vi "MoveAxes.vi"(0 "GoTo Array (Eng units all channels)":T5[](array[typedef]) {"Go To Position" step=100000.0}, 1 "Current Pulses In":dbl[](array[numeric]), 2 "Matched Configurations":T4(array[cluster]) {"Static Drive Configuration"."Indexer Mode  (FSA)" items=["Incremental", "Absolute"]; "Static Drive Configuration"."Buffer at Stop (SSH)" items=["Clear buffer", "Save and Continue"]; "Static Drive Configuration"."Buffer at Limit (SSG)" items=["Clear buffer", "Save and Continue"]; "Static Drive Configuration"."RS232 Echo Control (SSA)" items=["Echo ON", "Echo OFF"]; "Static Drive Configuration"."Reference edge of Home (OSH)" items=["CW", "CCW"]; "Static Drive Configuration"."Encoder Z for Home (OSD)" items=["Don't use", "Enable"]; "Static Drive Configuration"."Home Switch Sense (OSC)" items=["Normally Open", "Normally Closed"]; "Static Drive Configuration"."Home Position (OSB)" items=["Anywhere in Switch", "Edge of Switch"]; "Static Drive Configuration"."Limit Switch Sense (OSA)" items=["Normally Closed", "Normally Open"]; "Static Drive Configuration"."Limit Disable (LD)" items=["Both Enabled", "CW Disabled", "CCW Disabled", "Both Disabled"]; "Static Drive Configuration"."Stall Detect (FSH)" items=["Disable", "Enable"]; "Static Drive Configuration"."OP2 in Deadband (FSG)" items=["Don't Use", "ACTIVATE"]; "Static Drive Configuration"."Stop on Trigger 3 (FSF)" items=["Ignore", "STOP!"]; "Static Drive Configuration"."Activate OP1 on stall (FSE)" items=["Do not Activate", "ACTIVATE!"]; "Static Drive Configuration"."Stop on Stall (FSD)" items=["Continue", "STOP"]; "Static Drive Configuration"."Position Maintenance (FSC)" items=["Disabled", "Enabled"]; "Static Drive Configuration"."Step Mode  (FSB)" items=["Motor", "Encoder"]; "Static Drive Configuration"."Encoder Resolution (ER)" min=1 max=50000; "Static Drive Configuration"."Dead Band Window (DW)" min=0 max=999999999; "Static Drive Configuration"."Dead Band (DB)" min=0 max=999999999; "Static Drive Configuration"."Correction Gain % (CG)" items=["n/a", "12.5", "25", "37.5", "50", "62.5", "75", "87.5", "100"]; "Channel Properties"."Current Pos" format="%.2f"; "Channel Properties"."Backlash/Eng units" format="%.2f"; "Channel Properties"."Pulses/rev" format="%.2f"; "Channel Properties"."Pos Tolerance" format="%.2f"; "Channel Properties"."Pulses/unit" format="%.2f"; "Channel Properties"."Acc. Min" format="%.2f"; "Channel Properties"."Acc. Max" format="%.2f"; "Channel Properties"."Vel. Min" format="%.2f"; "Channel Properties"."Vel. Max" format="%.2f"; "Channel Properties"."Acc. Default" format="%.2f"; "Channel Properties"."Vel. Default" format="%.2f"}, 3 "Current Pos In":dbl[](array[numeric]) format="%.2f", 4 "Home":T1, 5 "Final move":bool) -> (6 "Current Pulses Out":dbl[](array[numeric]), 7 "Current Pos Out":dbl[](array[numeric]) format="%.2f", 8 "Error String":string)   [LabVIEW 2014]
uses:
  ~subVIs/DriveGotoCluster.ctl
  ~subVIs/DriveProperties.ctl
  ~subVIs/DriveStaticConfig.ctl
  Anemometry/Anemometry Sub Vis/Controls/Home.ctl
  ~subVIs/DriveClusterLower.ctl
  ~subVIs/GenericDriveCommand.ctl
  ~subVIs/DriveConfigGlobal.vi
panel:
  out "Retry number":i32
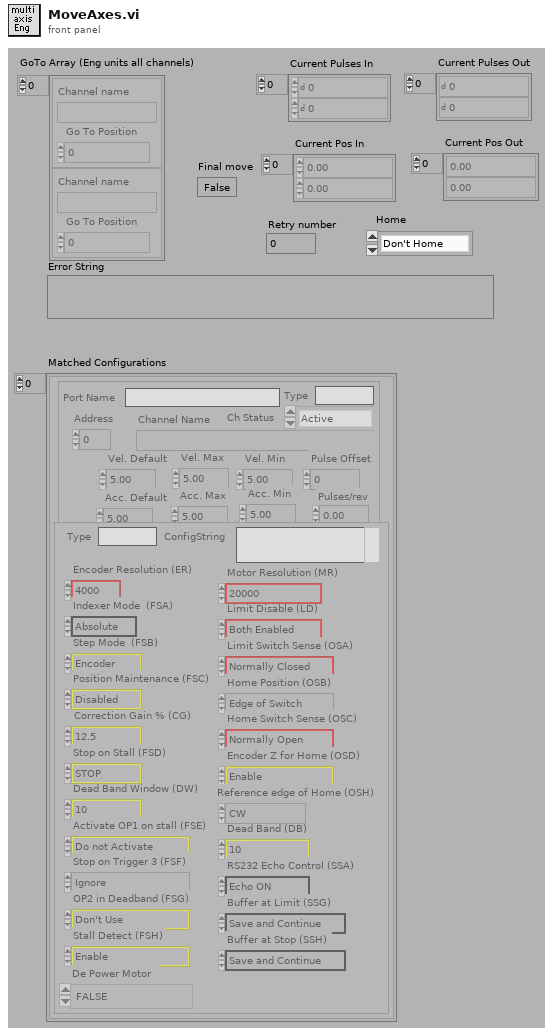
[diagram p1: front panel]
types:
  T1 = typedef "Home.ctl" = enum16{"Don't Home", "Home  +X", "Home  -X", "Home  +Y", "Home  -Y", "Home  +Z", "Home  -Z"}
  T2 = typedef "DriveProperties.ctl" = cluster{"Channel Name":string, "Vel. Default":dbl, "Acc. Default":dbl, "Vel. Max":dbl, "Vel. Min":dbl, "Acc. Max":dbl, "Acc. Min":dbl, "Pulses/unit":dbl, "Address":u8, "Pulse Offset":i32, "Pos Tolerance":dbl, "Pulses/rev":dbl, "Backlash/Eng units":dbl, "Current Pos":dbl, "Ch Status":enum16{"Active", "Offline", "Simulate"}, "Port Name":string, "Axis Transform mode":string, "Metadata Ch Name":string, "Type":string}
  T3 = typedef "DriveStaticConfig.ctl" = cluster{"Correction Gain % (CG)":u16, "Dead Band (DB)":i32, "Dead Band Window (DW)":i32, "Encoder Resolution (ER)":i32, "Step Mode  (FSB)":u16, "Position Maintenance (FSC)":u16, "Stop on Stall (FSD)":u16, "Activate OP1 on stall (FSE)":u16, "Stop on Trigger 3 (FSF)":u16, "OP2 in Deadband (FSG)":u16, "Stall Detect (FSH)":u16, "Limit Disable (LD)":u16, "Motor Resolution (MR)":enum16{"200", "400", "1000", "2000", "4000", "5000", "10000", "12800", "18000", "20000", "21600", "25000", "25400", "25600", "36000", "50000", "278528", "425984", "507904", "614400", "655360", "819200", "1024000"}, "Limit Switch Sense (OSA)":u16, "Home Position (OSB)":u16, "Home Switch Sense (OSC)":u16, "Encoder Z for Home (OSD)":u16, "Reference edge of Home (OSH)":u16, "RS232 Echo Control (SSA)":u16, "Buffer at Limit (SSG)":u16, "Buffer at Stop (SSH)":u16, "Indexer Mode  (FSA)":u16, "Type":string, "ConfigString":string, "De Power Motor":enum16{"TRUE", "FALSE"}}
  T4 = cluster{"Channel Properties":T2, "Static Drive Configuration":T3}[]
  T5 = typedef "DriveGotoCluster.ctl" = cluster{"Channel name":string, "Go To Position":dbl}
  T6 = typedef "GenericDriveCommand.ctl" = string
  T7 = cluster{"Channel Properties":T2, "Static Drive Configuration":T3}
  T8 = cluster{"Total travel time":dbl, "Accelaration time":dbl, "Accelation fractional distance":dbl}
  T9 = typedef "DriveClusterLower.ctl" = cluster{"Go To Position":dbl, "Velocity":dbl, "Acceleration":dbl, "Address":u8}
  T10 = typedef "AxisConfigCluster.ctl" = cluster{"Channel Properties":T2, "Static Drive Configuration":T3}
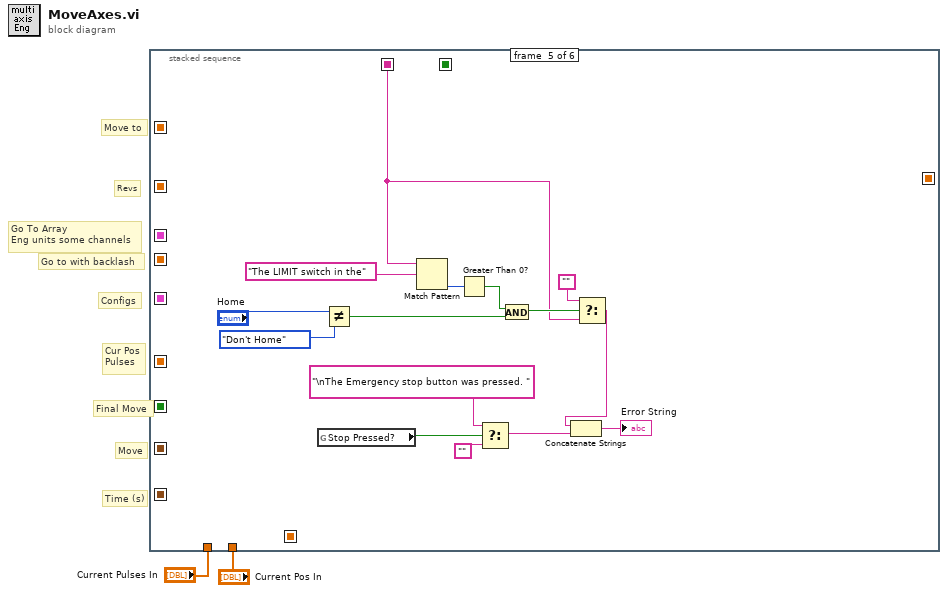
[diagram p0: block diagram]
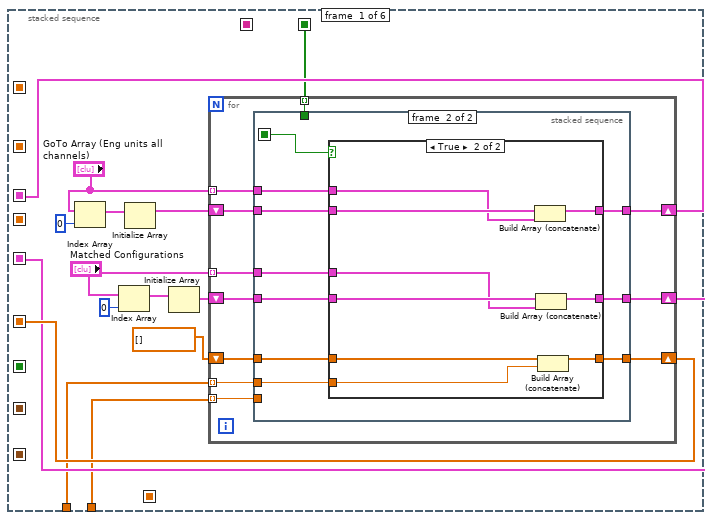
[diagram p2: hidden frame]
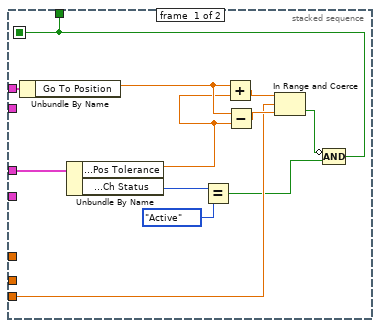
[diagram p3: hidden frame]
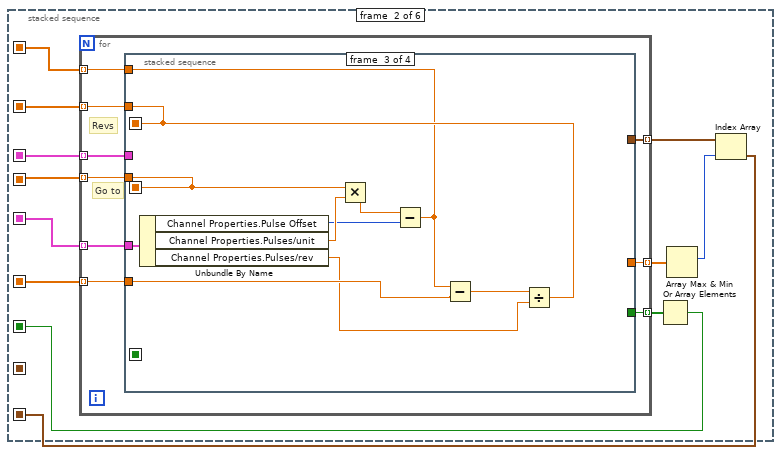
[diagram p5: hidden frame]
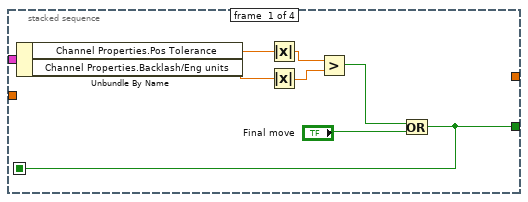
[diagram p6: hidden frame]
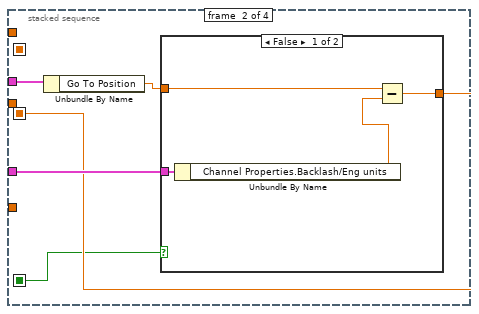
[diagram p7: hidden frame]
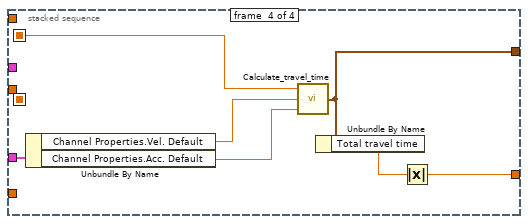
[diagram p9: hidden frame]
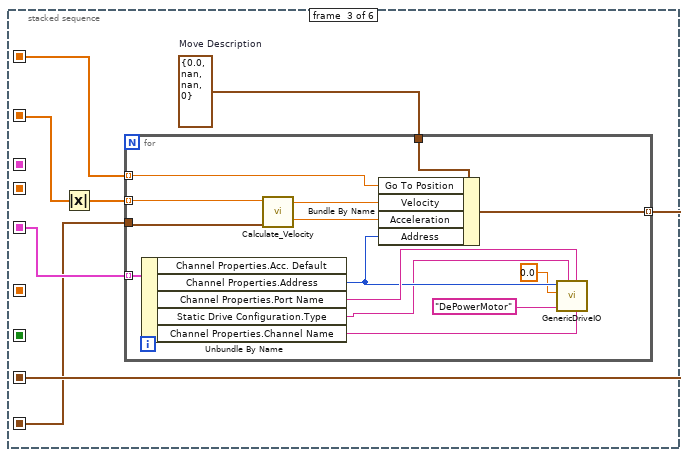
[diagram p10: hidden frame]
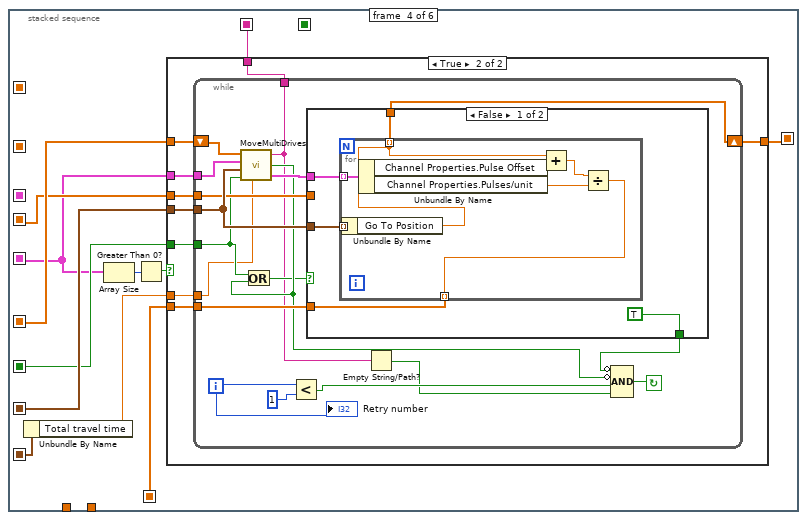
[diagram p11: hidden frame]
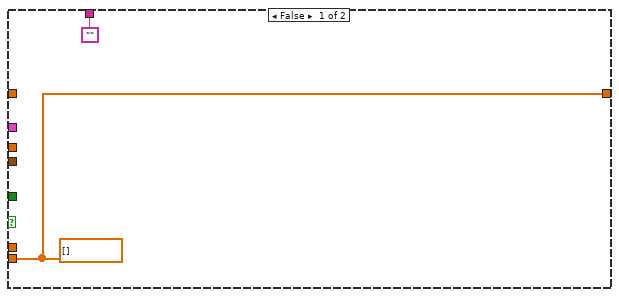
[diagram p12: hidden frame]
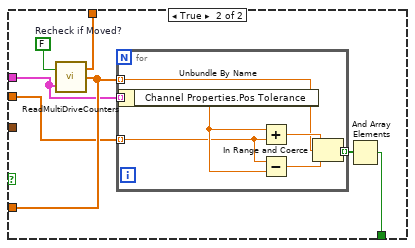
[diagram p13: hidden frame]
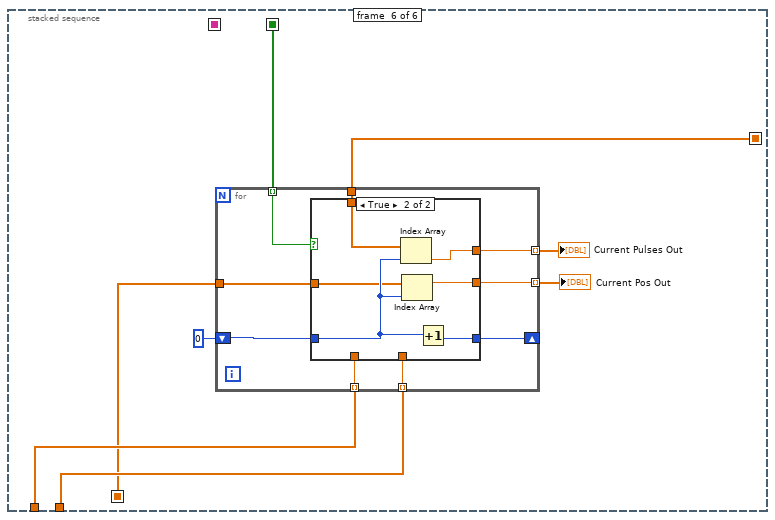
[diagram p14: hidden frame]
diagram:
  # "Go to with backlash"
  # "Final Move"
  # "Move"
  # "Cur Pos\nPulses"
  # "Configs"
  # "Go To Array\nEng units some channels"
  # "Revs"
  # "Move to"
  # "Time (s)"
  n1 = stacked-sequence {
    seq-local: [_ w63 _ _ _ _] -> [_ _ w119 w141 _ _]
    seq-local: [_ w73 _ _ _ _] -> [_ _ w124 _ _ _]
    seq-local: [_ w72 _ _ _ _] -> [_ _ w123 _ _ _]
    seq-local: [w7 _ _ _ _ _] -> [_ w70 _ _ _ _]
    seq-local: [w8 _ _ _ _ _] -> [_ w71 w122 w144 _ _]
    seq-local: [w9 _ _ _ _ _] -> [_ w69 _ w151 _ _]
    seq-local: [_ _ w121 _ _ _] -> [_ _ _ w150 _ _]
    seq-local: [_ _ _ w149 _ _] -> [_ _ _ _ _ w222]
    seq-local: [_ _ _ w148 _ _] -> [_ _ _ _ w212 _]
    seq-local: [w3 _ _ _ _ _] -> [_ _ _ _ _ w228]
    seq-local: [_ _ _ w147 _ _] -> [_ _ _ _ _ w223]
    seq-local: [_ w67 _ _ _ _] -> [_ _ _ w146 _ _]
    seq-local: [_ w66 _ _ _ _] -> [_ _ _ w145 _ _]
    tunnel: "Current Pulses In" -> [w5 _ _ _ _ w227]
    tunnel: "Current Pos In" -> [w4 _ _ _ _ w225]
    frame #0 {
      n2 = Index Array(array="GoTo Array (Eng units all channels)", index=0 ("Index")) -> (element=w15:T5)
      n3 = Index Array(array="Matched Configurations", index=0 ("Index")) -> (element=w13:T7)
      n4 = Initialize Array(w15) -> (w14:T5[])  [unwired: 1 out]
      n5 = Initialize Array(w13) -> (w10:T4)  [unwired: 1 out]
      n6 = for {
        tunnel: "Matched Configurations" -> [w28] mode=indexing
        tunnel: "GoTo Array (Eng units all channels)" -> [w27] mode=indexing
        tunnel: w4 -> [w26] mode=indexing
        shift-right: [w22] -> w7
        shift-left: w14 -> [w23]
        shift-right: [w24] -> w8
        shift-left: w10 -> [w25]
        shift-right: [w20] -> w9
        shift-left: dbl[] [] -> [w21]
        tunnel: w5 -> [w19] mode=indexing
        tunnel: [w18] -> w3 mode=indexing
        n7 = stacked-sequence {
          seq-local: [w33 _] -> [_ w50]
          tunnel: w28 -> [w39 w47]
          tunnel: w27 -> [w40 w44]
          tunnel: w26 -> [w35 _]
          tunnel: w25 -> [_ w49]
          tunnel: [_ w48] -> w24
          tunnel: w23 -> [_ w46]
          tunnel: [_ w45] -> w22
          tunnel: w21 -> [_ w43]
          tunnel: [_ w42] -> w20
          tunnel: w19 -> [_ w41]
          tunnel: [w33 _] -> w18
          frame #0 {
            n8 = Unbundle By Name(w40) -> ("Go To Position"=w38:dbl)
            n9 = Unbundle By Name(w39) -> ("Channel Properties.Pos Tolerance"=w32:dbl, "Channel Properties.Ch Status"=w31:enum16{"Active", "Offline", "Simulate"})
            n10 = Equal?(x=w31, y=enum16{"Active", "Offline", "Simulate"}."Active" ("Channel Properties.Ch Status")) -> (x = y?=w29:bool)
            n11 = Add(x=w38, y=w32) -> (x+y=w37:dbl)
            n12 = Subtract(x=w38, y=w32) -> (x-y=w36:dbl)
            n13 = In Range and Coerce(upper limit=w37, x=w35, lower limit=w36) -> (In Range?=w34:bool)  [unwired: 1 out]
            n14 = Compound Arithmetic op=AND(invert w34, w29) -> (w33:bool)
          }
          frame #1 {
            n15 = case shown="True" w50 {
              tunnel: w49 -> [w52 w62]
              tunnel: [w52 w61] -> w48
              tunnel: w47 -> [_ w60]
              tunnel: w46 -> [w53 w59]
              tunnel: [w53 w58] -> w45
              tunnel: w44 -> [_ w57]
              tunnel: w43 -> [w51 w56]
              tunnel: [w51 w55] -> w42
              tunnel: w41 -> [_ w54]
              frame False {
              }
              frame True {
                n16 = Build Array (concatenate)(w59, w57) -> (w58:T5[])
                n17 = Build Array (concatenate)(w62, w60) -> (w61:T4)
                n18 = Build Array (concatenate)(w56, w54) -> (w55:dbl[])
              }
            }
          }
        }
      }
    }
    frame #1 {
      n19 = for {
        tunnel: w71 -> [w83] mode=indexing
        tunnel: w70 -> [w82] mode=indexing
        tunnel: w69 -> [w81] mode=indexing
        tunnel: [w80] -> w74 mode=indexing
        tunnel: [w79] -> w73 mode=indexing
        tunnel: [w78] -> w72 mode=indexing
        tunnel: [w77] -> w68 mode=indexing
        tunnel: [w76] -> w66 mode=indexing
        tunnel: [w75] -> w65 mode=indexing
        # "Go to"
        # "Revs"
        n20 = stacked-sequence {
          seq-local: [_ _ w108 _] -> [_ _ _ w114]
          seq-local: [_ w93 _ _] -> [_ _ w102 _]
          seq-local: [w84 _ _ _] -> [_ w92 _ _]
          tunnel: w83 -> [w91 w95 w110 w118]
          tunnel: w82 -> [_ w96 _ _]
          tunnel: w81 -> [_ _ w109 _]
          tunnel: [_ _ _ w117] -> w80
          tunnel: [_ _ w105 _] -> w79
          tunnel: [_ _ w108 _] -> w78
          tunnel: [w84 _ _ _] -> w77
          tunnel: [_ _ w102 _] -> w76
          tunnel: [_ _ _ w113] -> w75
          frame #0 {
            n21 = Unbundle By Name(w91) -> ("Channel Properties.Pos Tolerance"=w90:dbl, "Channel Properties.Backlash/Eng units"=w89:dbl)
            n22 = Absolute Value(x=w90) -> (abs(x)=w88:dbl)
            n23 = Absolute Value(x=w89) -> (abs(x)=w87:dbl)
            n24 = Greater?(x=w88, y=w87) -> (0:w86:bool)
            n25 = Or(x=w86, y="Final move") -> (x .or. y?=w84:bool)
          }
          frame #1 {
            n26 = Unbundle By Name(w96) -> ("Go To Position"=w94:dbl)
            n27 = case shown="False" w92 {
              tunnel: w95 -> [w100 _]
              tunnel: w94 -> [w98 w101]
              tunnel: [w97 w101] -> w93
              frame False {
                n28 = Unbundle By Name(w100) -> ("Channel Properties.Backlash/Eng units"=w99:dbl)
                n29 = Subtract(x=w98, y=w99) -> (x-y=w97:dbl)
              }
              frame True {
              }
            }
          }
          frame #2 {
            n30 = Unbundle By Name(w110) -> ("Channel Properties.Pulse Offset"=w103:i32, "Channel Properties.Pulses/unit"=w111:dbl, "Channel Properties.Pulses/rev"=w106:dbl)
            n31 = Multiply(x=w102, y=w111) -> (x*y=w104:dbl)
            n32 = Subtract(x=w104, y=w103) -> (x-y=w105:dbl)
            n33 = Subtract(x=w105, y=w109) -> (x-y=w107:dbl)
            n34 = Divide(x=w107, y=w106) -> (x/y=w108:dbl)
          }
          frame #3 {
            n35 = Unbundle By Name(w118) -> ("Channel Properties.Vel. Default"=w115:dbl, "Channel Properties.Acc. Default"=w116:dbl)
            n36 = call "Calculate_travel_time.vi"("Default Acceleration"=w116, "Default Velocity"=w115, "Revs to travel"=w114) -> ("Times"=w113:T8)
            n37 = Unbundle By Name(w113) -> ("Total travel time"=w112:dbl)
            n38 = Absolute Value(x=w112) -> (abs(x)=w117:dbl)
          }
        }
      }
      n39 = Or Array Elements(Boolean array=w68) -> (logical OR=w67:bool)
      n40 = Array Max & Min(array=w74) -> (max index (indices)=w64:i32)  [unwired: 3 out]
      n41 = Index Array(array=w65, index=w64) -> (element=w63:T8)
    }
    frame #2 {
      w125 = T9 {"Go To Position"=0.0, "Velocity"=nan, "Acceleration"=nan, "Address"=0}  # Move Description
      n42 = Absolute Value(x=w123) -> (abs(x)=w120:dbl[])
      n43 = for {
        tunnel: w125 -> [w139]
        tunnel: w124 -> [w134] mode=indexing
        tunnel: w122 -> [w138] mode=indexing
        tunnel: w120 -> [w135] mode=indexing
        tunnel: [w137] -> w121 mode=indexing
        tunnel: w119 -> [w130]
        n44 = Unbundle By Name(w138) -> ("Channel Properties.Address"=w132:u8, "Channel Properties.Port Name"=w136:string, "Static Drive Configuration.Type"=w128:string, "Channel Properties.Channel Name"=w129:string)  [unwired: 1 out]
        n45 = call "Calculate_Velocity.vi"("Times"=w130, "Revs to travel"=w135) -> ("Acceleration"=w131:dbl, "Max Velocity"=w133:dbl)  [unwired: 1 in, 1 out]
        n46 = Bundle By Name(cluster=w139, "Go To Position"=w134, "Velocity"=w133, "Acceleration"=w131, "Address"=w132) -> (w137:T9)
        n47 = call "GenericDriveIO.vi"("GenericDriveCommand"=T6 "DePowerMotor", "Channel Name"=w129, "Numeric Value"=0.0, "Address"=w132, "Type"=w128, "Port Name"=w136) -> ()  [unwired: 1 in, 5 out]
      }
    }
    frame #3 {
      n48 = Unbundle By Name(w141) -> ("Total travel time"=w140:dbl)
      n49 = Array Size(array=w144) -> (size(s)=w143:i32)
      n50 = Greater Than 0?(x=w143) -> (x > 0?=w142:bool)
      n51 = case shown="True" w142 {
        tunnel: w151 -> [_ w162]
        tunnel: w144 -> [_ w161]
        tunnel: w150 -> [_ w160]
        tunnel: [w152 w159] -> w149
        tunnel: ["" w158] -> w148
        tunnel: [w152 w157] -> w147
        tunnel: w146 -> [_ w156]
        tunnel: w145 -> [_ w155]
        tunnel: w140 -> [_ w154]
        frame False {
          w152 = dbl[] [] ("Eng units")
        }
        frame True {
          n52 = while {
            tunnel: w154 -> [w163]
            tunnel: w155 -> [w170]
            tunnel: [w166] -> w158
            tunnel: w156 -> [w164]
            tunnel: [w175] -> w159
            shift-left: w162 -> [w178]
            shift-right: [w174] -> w157
            tunnel: w161 -> [w173]
            tunnel: w160 -> [w171]
            i -> [w180]
            stop <- w176 continue-if-true
            n53 = call "MoveMultiDrives.vi"("Start Counter"=w178, "Matched Configurations In"=w173, "GoTo Array (pulse position some channels)"=w171, "Final move"=w164, "Predicted Move Time"=w163) -> ("Error string"=w166:string, "Stop Pressed?"=w169:bool, "Matched Configurations Out"=w172:T10[])
            n54 = Or(x=w164, y=w169) -> (x .or. y?=w168:bool)
            n55 = Less?(x=w180, y=1) -> (x < y?=w177:bool)
            n56 = case shown="False" w168 {
              tunnel: w171 -> [w184 _]
              tunnel: [TRUE w199] -> w167
              tunnel: [w183 w198] -> w175
              tunnel: [w181 w197] -> w174
              tunnel: w172 -> [w182 w196]
              tunnel: w170 -> [_ w195]
              frame False {
                n57 = for {
                  tunnel: w184 -> [w192] mode=indexing
                  tunnel: [w189] -> w183 mode=indexing
                  tunnel: w182 -> [w191] mode=indexing
                  tunnel: [w187] -> w181 mode=indexing
                  n58 = Unbundle By Name(w192) -> ("Go To Position"=w187:dbl)
                  n59 = Unbundle By Name(w191) -> ("Channel Properties.Pulse Offset"=w188:i32, "Channel Properties.Pulses/unit"=w190:dbl)
                  n60 = Add(x=w187, y=w188) -> (x+y=w186:dbl)
                  n61 = Divide(x=w186, y=w190) -> (x/y=w189:dbl)
                }
              }
              frame True {
                w193 = FALSE  # Recheck if Moved?
                n62 = call "ReadMultiDriveCounters.vi"("Recheck if Moved?"=w193, "Matched Configurations"=w196) -> ("Pulses"=w197:dbl[], "Eng units"=w198:dbl[])  [unwired: 1 out]
                n63 = for {
                  tunnel: w195 -> [w200] mode=indexing
                  tunnel: [w206] -> w194 mode=indexing
                  tunnel: w198 -> [w202] mode=indexing
                  tunnel: w196 -> [w203] mode=indexing
                  n64 = Unbundle By Name(w203) -> ("Channel Properties.Pos Tolerance"=w201:dbl)
                  n65 = Add(x=w201, y=w200) -> (x+y=w205:dbl)
                  n66 = Subtract(x=w200, y=w201) -> (x-y=w204:dbl)
                  n67 = In Range and Coerce(upper limit=w205, x=w202, lower limit=w204) -> (In Range?=w206:bool)  [unwired: 1 out]
                }
                n68 = And Array Elements(Boolean array=w194) -> (logical AND=w199:bool)
              }
            }
            n69 = Empty String/Path?(string/path=w166) -> (empty?=w165:bool)
            n70 = Compound Arithmetic op=AND(invert w167, invert w169, w177, w165) -> (w176:bool)
            "Retry number" <- w180
          }
        }
      }
    }
    frame #4 {
      n71 = global read "DriveConfigGlobal.vi" "Stop Pressed?"() -> (w221:bool)
      n72 = Not Equal?(x="Home", y=Home."Don't Home" ("Home")) -> (x != y?=w207:bool)
      n73 = Match Pattern(string=w212, regular expression="The LIMIT switch in the") -> (offset past match=w215:i32)  [unwired: 1 in, 3 out]
      n74 = Greater Than 0?(x=w215) -> (x > 0?=w214:bool)
      n75 = Select(t="\nThe Emergency stop button was pressed. ", s=w221, f="") -> (s? t:f=w218:string)
      n76 = And(x=w214, y=w207) -> (x .and. y?=w213:bool)
      n77 = Select(t="", s=w213, f=w212) -> (s? t:f=w211:string)
      n78 = Concatenate Strings(w211, w218) -> (→"Error String":string)
    }
    frame #5 {
      n79 = for {
        shift-right: [w233] -> _
        shift-left: 0 -> [w232]
        tunnel: w228 -> [w238] mode=indexing
        tunnel: w227 -> [w237] mode=indexing
        tunnel: [w236] -> w226 mode=indexing
        tunnel: w225 -> [w235] mode=indexing
        tunnel: [w234] -> w224 mode=indexing
        tunnel: w223 -> [w231]
        tunnel: w222 -> [w230]
        n80 = case shown="True" w238 {
          tunnel: w237 -> [w241 _]
          tunnel: [w241 w245] -> w236
          tunnel: w235 -> [w240 _]
          tunnel: [w240 w244] -> w234
          tunnel: [w239 w247] -> w233
          tunnel: w232 -> [w239 w246]
          tunnel: w231 -> [_ w243]
          tunnel: w230 -> [_ w242]
          frame False {
          }
          frame True {
            n81 = Index Array(array=w243, index=w246) -> (element=w245:dbl)
            n82 = Index Array(array=w242, index=w246) -> (element=w244:dbl)
            n83 = Increment(x=w246) -> (x+1=w247:i32)
          }
        }
      }
      "Current Pulses Out" <- w226
      "Current Pos Out" <- w224
    }
  }
